vi "Write FGV Station No.vi"(8 "error in (no error)":errorcluster, 9 "Data":T1=enum."CurrentAction", 10 "String":string="3", 11 "AI in":refnum<class "AI.lvclass">) -> (0 "error out":errorcluster, 3 "AI out":refnum<class "AI.lvclass">)   [LabVIEW 2019, in "AI.lvclass"]
uses:
  AI.lvclass
  Ctrl/Auto Inspection Data Name.ctl
  Ctrl/Auto Inspection Station Name2.ctl
panel:
  in  "0Cv/1St":i32
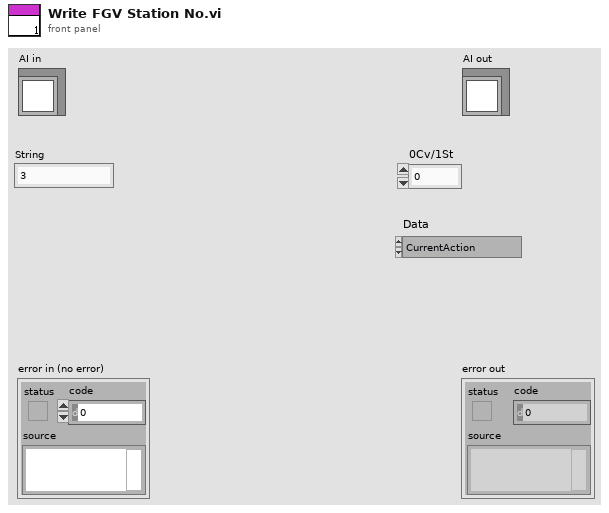
[diagram p1: front panel]
types:
  T1 = typedef "Auto Inspection Data Name.ctl" = enum16{"LocalRun", "ItemSN(TimeCode)", "CurrentAction", "Error", "Data", "OKNG", "電壓值", "電壓值判斷", "電流值", "電流值判斷", "Laser1 Data", "Laser2 Data", "Laser OKNG", "StationNO"}
  T2 = typedef "Auto Inspection Station Name2.ctl" = enum16{"S1Barcode", "S2Measure", "S3Measure", "S4Measure", "S5Measure", "S11_LaserCheck", "S8_Vision AI"}
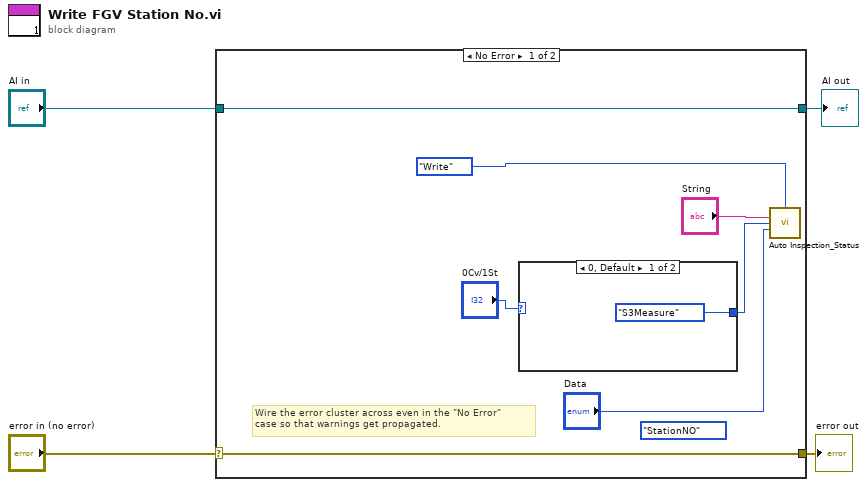
[diagram p0: block diagram]
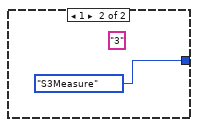
[diagram p2: hidden frame]
diagram:
  n1 = case shown="No Error" "error in (no error)" {
    selector: "error in (no error)" -> [w10 w15]
    tunnel: [w10 w15] -> w3
    tunnel: [w11 w14] -> w1
    tunnel: "AI in" -> [w11 w14]
    frame No Error {
      (unwired) Auto_Inspection_Data_Name."StationNO" ("Data")
      # "Wire the error cluster across even in the \"No Error\"\ncase so that warnings get propagated."
      n2 = case shown="0, Default" "0Cv/1St" {
        tunnel: [Auto_Inspection_Station_Name2."S3Measure" ("Station") Auto_Inspection_Station_Name2."S3Measure" ("Station")] -> w8
        frame 0, Default {
        }
        frame 1 {
          (unwired) "3"
        }
      }
      n3 = call "Auto Inspection_Status.vi"("Action"=enum16{"Initial", "Write", "Read"}."Write", "DataIn"="String", "Station"=w8, "Data"="Data") -> ()  [unwired: 9 in, 3 out]
    }
    frame Error {
    }
  }
  "error out" <- w3
  "AI out" <- w1
